vi "Set Boolean Box Properties using Property Node.vi"(0 "Game Board Cluster reference":refnum<vi>, 1 "Boolean Text Control States":T2, 5 "Array - In":dbl[][](array[numeric]), 7 "Current State":T1, 11 "error in (no error)":errorcluster) -> (6 "Array - Out":dbl[][](array[numeric]), 15 "error out":errorcluster)   [LabVIEW 2021]
uses:
  Controls/Boolean Text Control States.ctl
  Controls/State.ctl
  <vilib>/Utility/miscctls.llb/LVTextColorsTypeDef.ctl
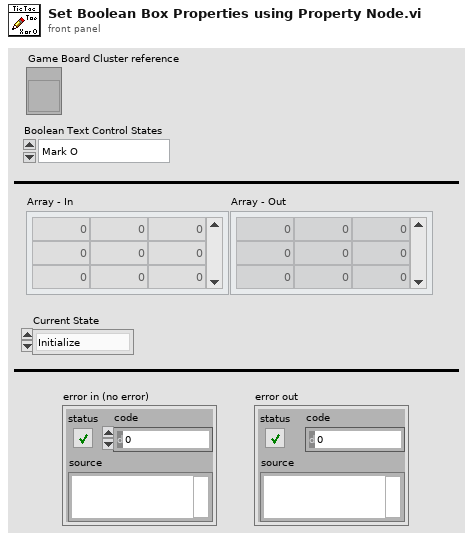
[diagram p1: front panel]
types:
  T1 = typedef "State.ctl" = enum16{"Initialize", "Wait for Event", "Set Left Upp", "Set Left Mid", "Set Left Bot", "Set Middle Upp", "Set Middle Mid", "Set Middle Bot", "Set Right Upp", "Set Right Mid", "Set Right Bot", "Check Game Status", "Exit"}
  T2 = typedef "Boolean Text Control States.ctl" = enum16{"Mark O", "Mark X", "Strike-through O", "Strike-through X"}
  T3 = typedef "LVTextColorsTypeDef.ctl" = cluster{"Text Color":u32, "Background Color":u32}
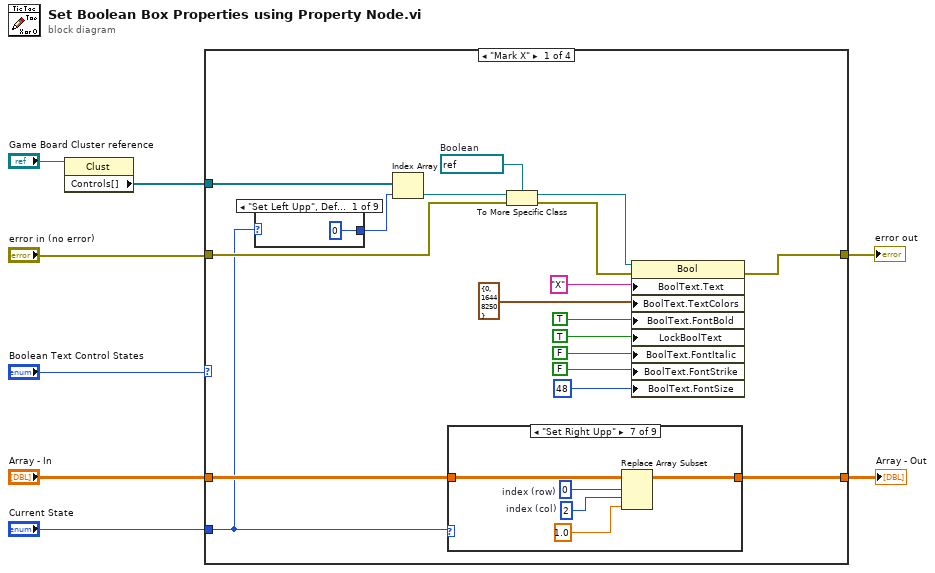
[diagram p0: block diagram]
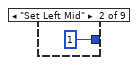
[diagram p2: hidden frame]
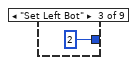
[diagram p3: hidden frame]
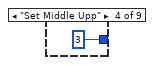
[diagram p4: hidden frame]
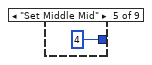
[diagram p5: hidden frame]
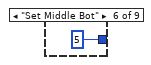
[diagram p6: hidden frame]
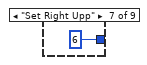
[diagram p7: hidden frame]
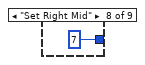
[diagram p8: hidden frame]
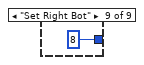
[diagram p9: hidden frame]
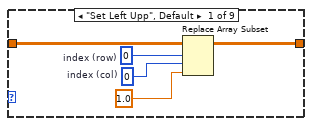
[diagram p10: hidden frame]
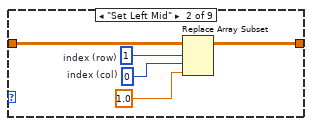
[diagram p11: hidden frame]
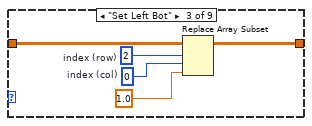
[diagram p12: hidden frame]
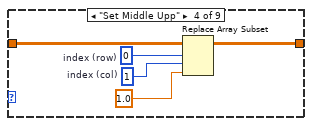
[diagram p13: hidden frame]
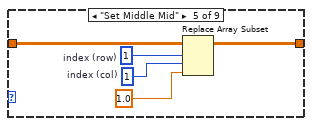
[diagram p14: hidden frame]
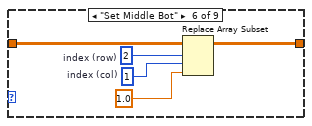
[diagram p15: hidden frame]
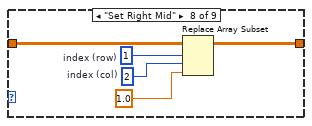
[diagram p16: hidden frame]
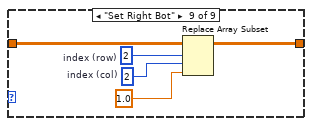
[diagram p17: hidden frame]
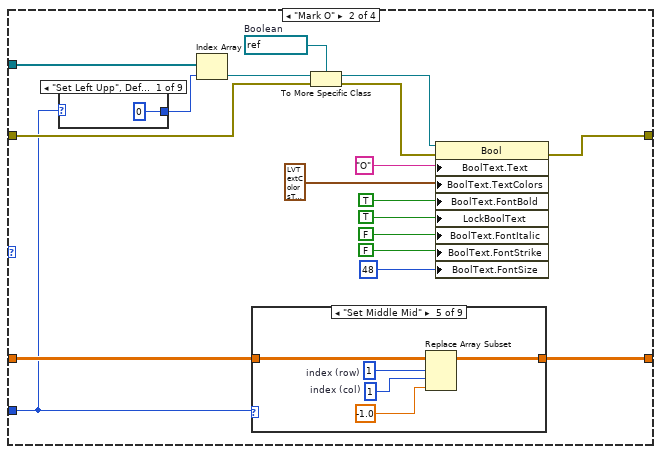
[diagram p18: hidden frame]
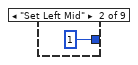
[diagram p19: hidden frame]
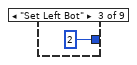
[diagram p20: hidden frame]
diagram:
  n1 = property class="Clust"(reference="Game Board Cluster reference") -> ("Controls[]"=w1:refnum<vi>[])  [unwired: 1 in, 2 out]
  n2 = case shown="\"Mark X\"" "Boolean Text Control States" {
    tunnel: [w19 w91 w162 w188] -> w6
    tunnel: "error in (no error)" -> [w12 w84 w158 w184]
    tunnel: "Array - In" -> [w18 w90 w154 w180]
    tunnel: "Current State" -> [w10 w82 w153 w179]
    tunnel: [w17 w89 w154 w180] -> w3
    tunnel: w1 -> [w14 w86 w157 w183]
    frame "Mark X" {
      w15 = refnum<vi> refnum  # Boolean
      n3 = case shown="\"Set Left Upp\", Default" w10 {
        tunnel: [0 ("index") 1 ("index") 2 ("index") 3 ("index") 4 ("index") 5 ("index") 6 ("index") 7 ("index") 8 ("index")] -> w9
        frame "Set Left Upp", Default {
        }
        frame "Set Left Mid" {
        }
        frame "Set Left Bot" {
        }
        frame "Set Middle Upp" {
        }
        frame "Set Middle Mid" {
        }
        frame "Set Middle Bot" {
        }
        frame "Set Right Upp" {
        }
        frame "Set Right Mid" {
        }
        frame "Set Right Bot" {
        }
      }
      n4 = Index Array(array=w14, index=w9) -> (element=w16:refnum<vi>)
      n5 = case shown="\"Set Right Upp\"" w10 {
        tunnel: w18 -> [w40 w45 w50 w55 w60 w65 w70 w75 w80]
        tunnel: [w38 w43 w48 w53 w58 w63 w68 w73 w78] -> w17
        frame "Set Left Upp", Default {
          w37 = 0  # index (col)
          w39 = 0  # index (row)
          n6 = Replace Array Subset(array=w40, new element=1.0 ("new element/subarray"), index (row)=w39, index (col)=w37) -> (w38:dbl[][])
        }
        frame "Set Left Mid" {
          w42 = 0  # index (col)
          w44 = 1  # index (row)
          n7 = Replace Array Subset(array=w45, new element=1.0 ("new element/subarray"), index (row)=w44, index (col)=w42) -> (w43:dbl[][])
        }
        frame "Set Left Bot" {
          w47 = 0  # index (col)
          w49 = 2  # index (row)
          n8 = Replace Array Subset(array=w50, new element=1.0 ("new element/subarray"), index (row)=w49, index (col)=w47) -> (w48:dbl[][])
        }
        frame "Set Middle Upp" {
          w52 = 1  # index (col)
          w54 = 0  # index (row)
          n9 = Replace Array Subset(array=w55, new element=1.0 ("new element/subarray"), index (row)=w54, index (col)=w52) -> (w53:dbl[][])
        }
        frame "Set Middle Mid" {
          w57 = 1  # index (col)
          w59 = 1  # index (row)
          n10 = Replace Array Subset(array=w60, new element=1.0 ("new element/subarray"), index (row)=w59, index (col)=w57) -> (w58:dbl[][])
        }
        frame "Set Middle Bot" {
          w62 = 1  # index (col)
          w64 = 2  # index (row)
          n11 = Replace Array Subset(array=w65, new element=1.0 ("new element/subarray"), index (row)=w64, index (col)=w62) -> (w63:dbl[][])
        }
        frame "Set Right Upp" {
          w67 = 2  # index (col)
          w69 = 0  # index (row)
          n12 = Replace Array Subset(array=w70, new element=1.0 ("new element/subarray"), index (row)=w69, index (col)=w67) -> (w68:dbl[][])
        }
        frame "Set Right Mid" {
          w72 = 2  # index (col)
          w74 = 1  # index (row)
          n13 = Replace Array Subset(array=w75, new element=1.0 ("new element/subarray"), index (row)=w74, index (col)=w72) -> (w73:dbl[][])
        }
        frame "Set Right Bot" {
          w77 = 2  # index (col)
          w79 = 2  # index (row)
          n14 = Replace Array Subset(array=w80, new element=1.0 ("new element/subarray"), index (row)=w79, index (col)=w77) -> (w78:dbl[][])
        }
      }
      n15 = To More Specific Class(target class=w15, reference=w16, error in=w12) -> (specific class reference=w13:refnum<vi>, error out=w11:errorcluster)
      n16 = property on="Property Node" class="Bool"(reference=w13, error in=w11, "BoolText.Text"="X" ("Boolean Text.Text"), "BoolText.TextColors"=T3 {"Text Color"=0, "Background Color"=16448250} ("Boolean Text.Text Colors"), "BoolText.FontBold"=TRUE ("Boolean Text.Font:Bold"), "LockBoolText"=TRUE ("Lock Boolean Text In Center"), "BoolText.FontItalic"=FALSE ("Boolean Text.Font:Italic"), "BoolText.FontStrike"=FALSE ("Boolean Text.Font:Strikeout"), "BoolText.FontSize"=u32 48 ("Boolean Text.Font:Size")) -> (error out=w19:errorcluster)  [unwired: 1 out]
    }
    frame "Mark O" {
      w87 = refnum<vi> refnum  # Boolean
      n17 = case shown="\"Set Left Upp\", Default" w82 {
        tunnel: [0 ("index") 1 ("index") 2 ("index") 3 ("index") 4 ("index") 5 ("index") 6 ("index") 7 ("index") 8 ("index")] -> w81
        frame "Set Left Upp", Default {
        }
        frame "Set Left Mid" {
        }
        frame "Set Left Bot" {
        }
        frame "Set Middle Upp" {
        }
        frame "Set Middle Mid" {
        }
        frame "Set Middle Bot" {
        }
        frame "Set Right Upp" {
        }
        frame "Set Right Mid" {
        }
        frame "Set Right Bot" {
        }
      }
      n18 = Index Array(array=w86, index=w81) -> (element=w88:refnum<vi>)
      n19 = case shown="\"Set Middle Mid\"" w82 {
        tunnel: w90 -> [w112 w117 w122 w127 w132 w137 w142 w147 w152]
        tunnel: [w110 w115 w120 w125 w130 w135 w140 w145 w150] -> w89
        frame "Set Left Upp", Default {
          w109 = 0  # index (col)
          w111 = 0  # index (row)
          n20 = Replace Array Subset(array=w112, new element=-1.0 ("new element/subarray"), index (row)=w111, index (col)=w109) -> (w110:dbl[][])
        }
        frame "Set Left Mid" {
          w114 = 0  # index (col)
          w116 = 1  # index (row)
          n21 = Replace Array Subset(array=w117, new element=-1.0 ("new element/subarray"), index (row)=w116, index (col)=w114) -> (w115:dbl[][])
        }
        frame "Set Left Bot" {
          w119 = 0  # index (col)
          w121 = 2  # index (row)
          n22 = Replace Array Subset(array=w122, new element=-1.0 ("new element/subarray"), index (row)=w121, index (col)=w119) -> (w120:dbl[][])
        }
        frame "Set Middle Upp" {
          w124 = 1  # index (col)
          w126 = 0  # index (row)
          n23 = Replace Array Subset(array=w127, new element=-1.0 ("new element/subarray"), index (row)=w126, index (col)=w124) -> (w125:dbl[][])
        }
        frame "Set Middle Mid" {
          w129 = 1  # index (col)
          w131 = 1  # index (row)
          n24 = Replace Array Subset(array=w132, new element=-1.0 ("new element/subarray"), index (row)=w131, index (col)=w129) -> (w130:dbl[][])
        }
        frame "Set Middle Bot" {
          w134 = 1  # index (col)
          w136 = 2  # index (row)
          n25 = Replace Array Subset(array=w137, new element=-1.0 ("new element/subarray"), index (row)=w136, index (col)=w134) -> (w135:dbl[][])
        }
        frame "Set Right Upp" {
          w139 = 2  # index (col)
          w141 = 0  # index (row)
          n26 = Replace Array Subset(array=w142, new element=-1.0 ("new element/subarray"), index (row)=w141, index (col)=w139) -> (w140:dbl[][])
        }
        frame "Set Right Mid" {
          w144 = 2  # index (col)
          w146 = 1  # index (row)
          n27 = Replace Array Subset(array=w147, new element=-1.0 ("new element/subarray"), index (row)=w146, index (col)=w144) -> (w145:dbl[][])
        }
        frame "Set Right Bot" {
          w149 = 2  # index (col)
          w151 = 2  # index (row)
          n28 = Replace Array Subset(array=w152, new element=-1.0 ("new element/subarray"), index (row)=w151, index (col)=w149) -> (w150:dbl[][])
        }
      }
      n29 = To More Specific Class(target class=w87, reference=w88, error in=w84) -> (specific class reference=w85:refnum<vi>, error out=w83:errorcluster)
      n30 = property on="Property Node" class="Bool"(reference=w85, error in=w83, "BoolText.Text"="O" ("Boolean Text.Text"), "BoolText.TextColors"=T3 {"Text Color"=16711680, "Background Color"=16448250} ("Boolean Text.Text Colors"), "BoolText.FontBold"=TRUE ("Boolean Text.Font:Bold"), "LockBoolText"=TRUE ("Lock Boolean Text In Center"), "BoolText.FontItalic"=FALSE ("Boolean Text.Font:Italic"), "BoolText.FontStrike"=FALSE ("Boolean Text.Font:Strikeout"), "BoolText.FontSize"=u32 48 ("Boolean Text.Font:Size")) -> (error out=w91:errorcluster)  [unwired: 1 out]
    }
    frame "Strike-through X" {
      w160 = refnum<vi> refnum  # Boolean
      n31 = case shown="\"Set Left Upp\", Default" w153 {
        tunnel: [0 ("index") 1 ("index") 2 ("index") 3 ("index") 4 ("index") 5 ("index") 6 ("index") 7 ("index") 8 ("index")] -> w159
        frame "Set Left Upp", Default {
        }
        frame "Set Left Mid" {
        }
        frame "Set Left Bot" {
        }
        frame "Set Middle Upp" {
        }
        frame "Set Middle Mid" {
        }
        frame "Set Middle Bot" {
        }
        frame "Set Right Upp" {
        }
        frame "Set Right Mid" {
        }
        frame "Set Right Bot" {
        }
      }
      n32 = Index Array(array=w157, index=w159) -> (element=w161:refnum<vi>)
      n33 = To More Specific Class(target class=w160, reference=w161, error in=w158) -> (specific class reference=w155:refnum<vi>, error out=w156:errorcluster)
      n34 = property on="Property Node" class="Bool"(reference=w155, error in=w156, "BoolText.Text"="X" ("Boolean Text.Text"), "BoolText.TextColors"=T3 {"Text Color"=0, "Background Color"=16448250} ("Boolean Text.Text Colors"), "BoolText.FontBold"=TRUE ("Boolean Text.Font:Bold"), "LockBoolText"=TRUE ("Lock Boolean Text In Center"), "BoolText.FontItalic"=FALSE ("Boolean Text.Font:Italic"), "BoolText.FontStrike"=TRUE ("Boolean Text.Font:Strikeout"), "BoolText.FontSize"=u32 48 ("Boolean Text.Font:Size")) -> (error out=w162:errorcluster)  [unwired: 1 out]
    }
    frame "Strike-through O" {
      w186 = refnum<vi> refnum  # Boolean
      n35 = case shown="\"Set Left Upp\", Default" w179 {
        tunnel: [0 ("index") 1 ("index") 2 ("index") 3 ("index") 4 ("index") 5 ("index") 6 ("index") 7 ("index") 8 ("index")] -> w185
        frame "Set Left Upp", Default {
        }
        frame "Set Left Mid" {
        }
        frame "Set Left Bot" {
        }
        frame "Set Middle Upp" {
        }
        frame "Set Middle Mid" {
        }
        frame "Set Middle Bot" {
        }
        frame "Set Right Upp" {
        }
        frame "Set Right Mid" {
        }
        frame "Set Right Bot" {
        }
      }
      n36 = Index Array(array=w183, index=w185) -> (element=w187:refnum<vi>)
      n37 = To More Specific Class(target class=w186, reference=w187, error in=w184) -> (specific class reference=w181:refnum<vi>, error out=w182:errorcluster)
      n38 = property on="Property Node" class="Bool"(reference=w181, error in=w182, "BoolText.Text"="O" ("Boolean Text.Text"), "BoolText.TextColors"=T3 {"Text Color"=16711680, "Background Color"=16448250} ("Boolean Text.Text Colors"), "BoolText.FontBold"=TRUE ("Boolean Text.Font:Bold"), "LockBoolText"=TRUE ("Lock Boolean Text In Center"), "BoolText.FontItalic"=FALSE ("Boolean Text.Font:Italic"), "BoolText.FontStrike"=TRUE ("Boolean Text.Font:Strikeout"), "BoolText.FontSize"=u32 48 ("Boolean Text.Font:Size")) -> (error out=w188:errorcluster)  [unwired: 1 out]
    }
  }
  "error out" <- w6
  "Array - Out" <- w3
